vi "GetHeadPropertiesAttributesFromConfigDict.vi"(8 "error in (no error)":errorcluster, 10 "Head":T2=enum."1", 11 "TopLevel in":refnum<class "TopLevel.lvclass">) -> (0 "error out":errorcluster, 1 "found":bool, 2 "#attributes":T1, 3 "TopLevel out":refnum<class "TopLevel.lvclass">)   [LabVIEW 2022 SP3, in "TopLevel.lvclass"]
uses:
  TopLevel.lvclass
  Typedefs/PrinterHeads--Enum.ctl
  Common/Controls/DLPConfig)Init_HeadPropertyAttr--Cluster.ctl
  DLP2/DataTypes/DLP2_PrinterHeadProperties.ctl
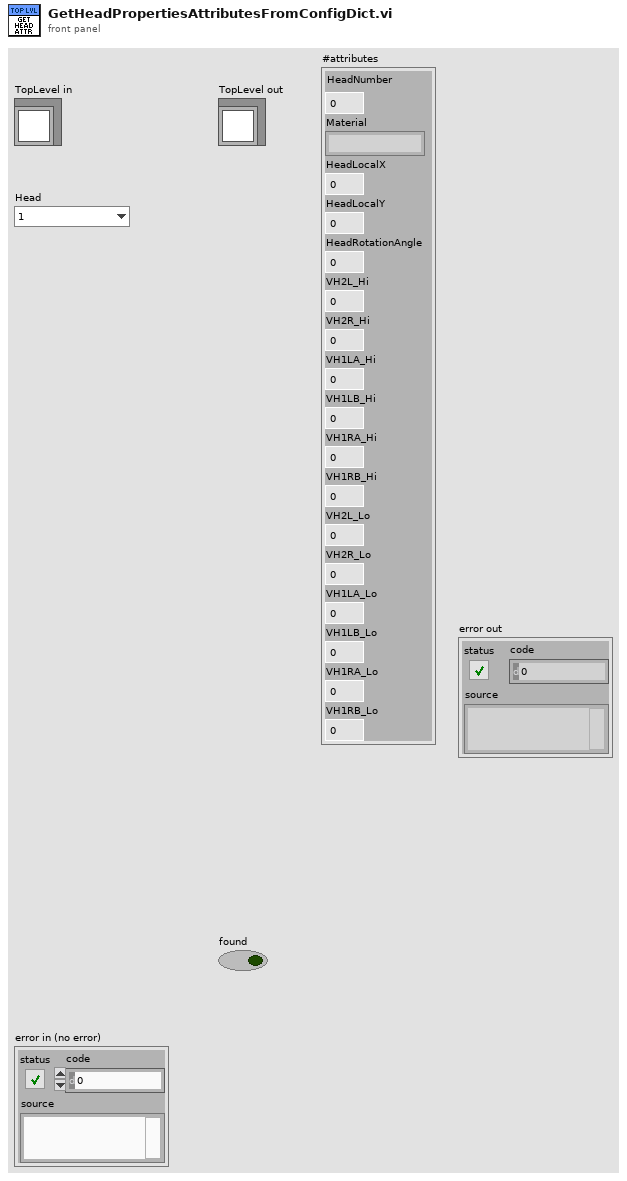
[diagram p1: front panel]
types:
  T1 = typedef "DLPConfig)Init_HeadPropertyAttr--Cluster.ctl" = cluster{"HeadNumber":u8, "Material":string, "HeadLocalX":dbl, "HeadLocalY":dbl, "HeadRotationAngle":dbl, "VH2L_Hi":dbl, "VH2R_Hi":dbl, "VH1LA_Hi":dbl, "VH1LB_Hi":dbl, "VH1RA_Hi":dbl, "VH1RB_Hi":dbl, "VH2L_Lo":dbl, "VH2R_Lo":dbl, "VH1LA_Lo":dbl, "VH1LB_Lo":dbl, "VH1RA_Lo":dbl, "VH1RB_Lo":dbl}
  T2 = typedef "PrinterHeads--Enum.ctl" = enum16{"-1", "1", "2", "3", "4", "5", "6"}
  T3 = typedef "DLP2_PrinterHeadProperties.ctl" = cluster{"#attributes":T1}
  T4 = typedef "TD Dynamic CVT DVR--ref.ctl" = refnum<data-value>
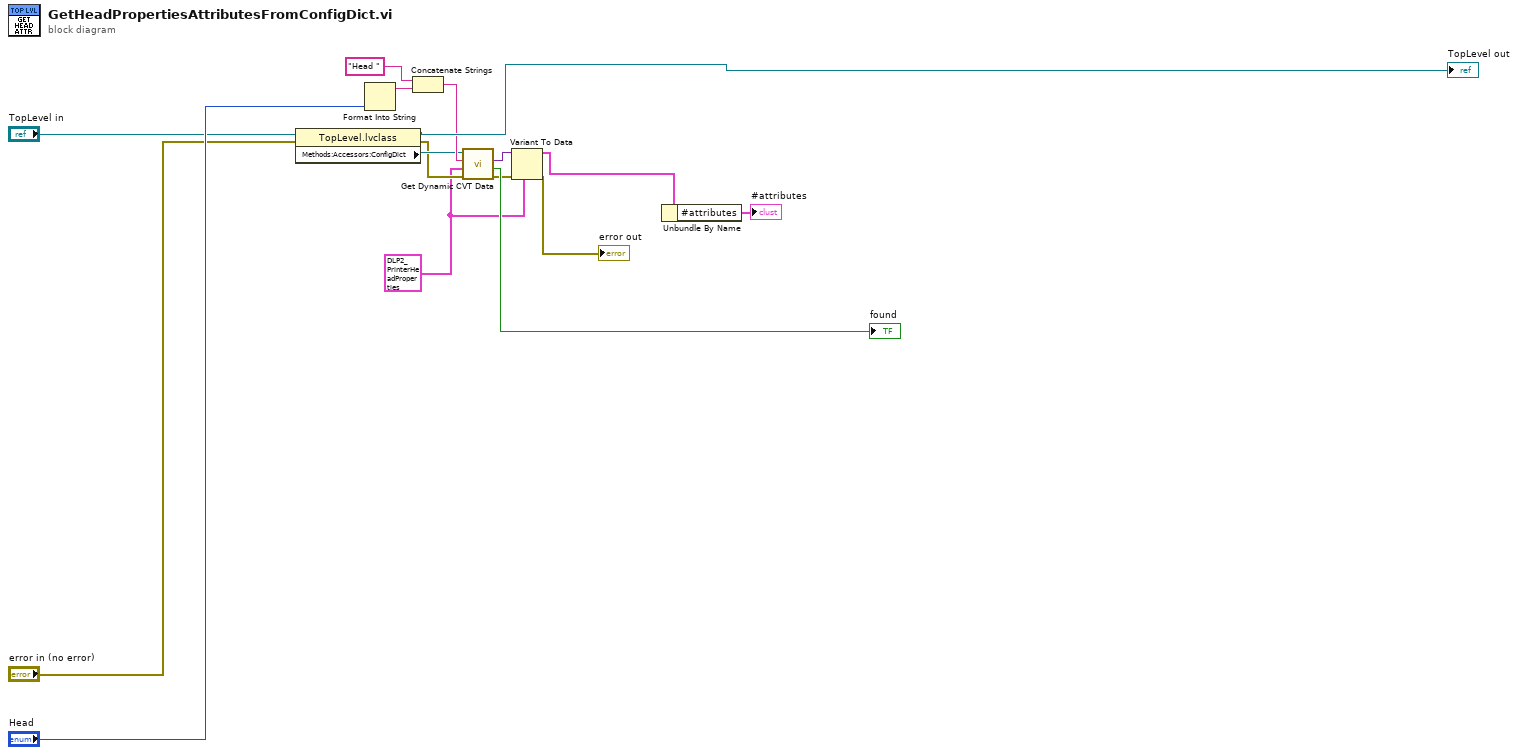
[diagram p0: block diagram]
diagram:
  w3 = T3 {"#attributes"={"HeadNumber"=0, "Material"="", "HeadLocalX"=0.0, "HeadLocalY"=0.0, "HeadRotationAngle"=0.0, "VH2L_Hi"=0.0, "VH2R_Hi"=0.0, "VH1LA_Hi"=0.0, "VH1LB_Hi"=0.0, "VH1RA_Hi"=0.0, "VH1RB_Hi"=0.0, "VH2L_Lo"=0.0, "VH2R_Lo"=0.0, "VH1LA_Lo"=0.0, "VH1LB_Lo"=0.0, "VH1RA_Lo"=0.0, "VH1RB_Lo"=0.0}}
  n1 = property class="TopLevel.lvclass"(reference="TopLevel in", error in="error in (no error)") -> (reference out=→"TopLevel out":refnum<class "TopLevel.lvclass">, error out=w4:errorcluster, "Methods:Accessors:ConfigDict"=w8:T4)
  n2 = Format Into String("Head") -> (resulting string=w10:string)  [unwired: 3 in, 1 out]
  n3 = Concatenate Strings("Head " ("string"), w10) -> (w12:string)
  n4 = call <vilib>:"Get Dynamic CVT Data.vi"("error in (no error)"=w4, "default value (empty variant)"=w3, "DataName"=w12, "dCVT DVR"=w8) -> ("error out"=w13:errorcluster, "found"=→"found":bool, "value"=w14:variant)  [unwired: 4 in, 1 out]
  n5 = Variant To Data(error in=w13, type=w3, Variant=w14) -> (data=w2:T3, error out=→"error out":errorcluster)
  n6 = Unbundle By Name(w2) -> ("#attributes"=→"#attributes":T1)
